vi "Application_GetExistingComports.vi"(8 "error in (no error)":errorcluster) -> (0 "error out":errorcluster, 2 "Comport":string[](array[string]), 3 "Registry Name":string[](array[string]))   [LabVIEW 2016]
doc: "Queries the Windows Registy for ComPorts since VISA resources are too slow in updating disconnected ComPorts.\n\nAndreas Elmiger, 05.01.2017"
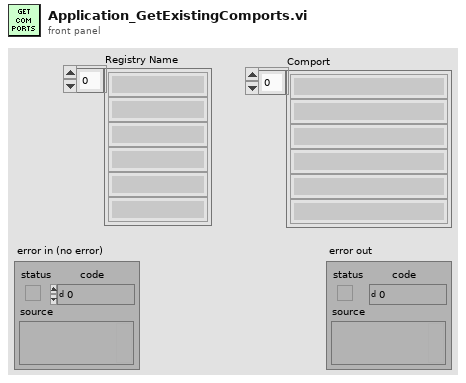
[diagram p1: front panel]
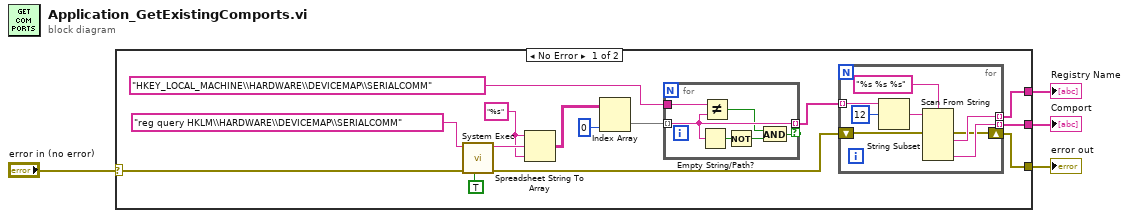
[diagram p0: block diagram]
diagram:
  n1 = case shown="No Error" "error in (no error)" {
    selector: "error in (no error)" -> [w5 w33]
    tunnel: [w11 _] -> w4
    tunnel: [w10 _] -> w3
    tunnel: [w6 w33] -> w2
    frame No Error {
      w16 = "%s" ("format string")
      n2 = call <vilib>:"System Exec.vi"("run minimized? (F)"=TRUE, "error in (no error)"=w5, "command line"="reg query HKLM\\HARDWARE\\DEVICEMAP\\SERIALCOMM") -> ("error out"=w7:errorcluster, "standard output"=w17:string)  [unwired: 5 in, 2 out]
      n3 = Spreadsheet String To Array(format string=w16, spreadsheet string=w17, array type (2D Dbl)=w16) -> (array=w15:string[][])  [unwired: 1 in]
      n4 = Index Array(array=w15, index (col)=0 ("disabled index (col)")) -> (element=w13:string[])  [unwired: 1 in]
      n5 = for {
        tunnel: w13 -> [w30] mode=indexing
        tunnel: [w30] -> w12 mode=indexing if=w28
        tunnel: "HKEY_LOCAL_MACHINE\\HARDWARE\\DEVICEMAP\\SERIALCOMM" ("format string") -> [w29]
        n6 = Empty String/Path?(string/path=w30) -> (empty?=w32:bool)
        n7 = Not Equal?(x=w29, y=w30) -> (x != y?=w27:bool)
        n8 = Not(x=w32) -> (.not. x?=w31:bool)
        n9 = And(x=w27, y=w31) -> (x .and. y?=w28:bool)
      }
      n10 = for {
        tunnel: w12 -> [w26] mode=indexing
        tunnel: [w22] -> w10 mode=indexing
        tunnel: [w21] -> w11 mode=indexing
        shift-right: [w19] -> w6
        shift-left: w7 -> [w20]
        n11 = String Subset(string=w26, offset (0)=12) -> (substring=w24:string)  [unwired: 1 in]
        n12 = Scan From String(format string="%s %s %s", input string=w24, error in=w20) -> (error out=w19:errorcluster, output 1=w22:string, output 3=w21:string)  [unwired: 5 in, 2 out]
      }
    }
    frame Error {
    }
  }
  "Registry Name" <- w3
  "Comport" <- w4
  "error out" <- w2
